vi "Simple edge timing.vi"() -> ()   [LabVIEW 2018]
uses:
  <vilib>/Platform/TimedLoop/XDataNode/timing_clust.ctl
  <vilib>/Platform/TimedLoop/XDataNode/nitl_modes.ctl
  <vilib>/Platform/TimedLoop/XDataNode/wakeup.ctl
  <vilib>/rvi/Emulation/niFpgaSctlEmulationGetInTimedLoop.vi
  <vilib>/rvi/Emulation/niFpgaProcessEmulError.vi
  <vilib>/rvi/Emulation/niFpgaEmulationReportErrorSimple.vi
  <vilib>/rvi/Emulation/niFpgaGetClockAttributes.vi
  <vilib>/rvi/Emulation/niFpgaCriticalErrorInLSC.vi
  <vilib>/rvi/eio/common/nirviEmuTemplateMethod_errors.vi
  <vilib>/platform/TimedLoop/XDataNode/XDataNode.xnode
  <vilib>/eio/EIONode/EIONode.xnode
  <vilib>/Platform/TimedLoop/XDataNode/XDNodeRunTimeDep.lvlib
panel:
  in  "STOP":bool
  out "pulses":u32 caption="Clock cycles"
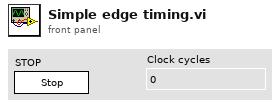
[diagram p1: front panel]
types:
  T1 = typedef "XDNodeRunTimeDep.lvlib/timing_clust.ctl" = cluster{"Expected End [f-1]":u64, "Actual End [f-1]":u64, "Finished Late? [f-1]":bool, "Expected End [i-1]":u64, "Actual End [i-1]":u64, "Finished Late? [i-1]":bool, "Expected Start [i]":u64, "Actual Start [i]":u64, "Expected Start [f]":u64, "Actual Start [f]":u64, "Source Name":string, "Structure Name":string, "Period":i64, "Deadline":i64, "Offset":i64, "Start":i64, "Priority":i32, "Timeout":i32, "Mode":T2, "Wakeup Reason":T3, "Error":errorcluster, "Source Type":string, "Secondary Source Type":string, "Global End Time":u64, "Global Start Time":u64, "Frame Duration":u64, "Iteration Duration":u64, "Assigned CPU":i32, "I/O Scan Engine Mode":u32}
  T2 = typedef "XDNodeRunTimeDep.lvlib/nitl_modes.ctl" = enum32{"No Change", "Process missed periods, maintain original phase", "Discard missed periods, maintain original phase", "Process missed periods, ignore original phase", "Discard missed periods, ignore original phase"}
  T3 = typedef "XDNodeRunTimeDep.lvlib/wakeup.ctl" = enum32{"Normal", "Aborted", "Asynchronous wakeup", "Timing source error", "Timed loop error", "Timeout"}
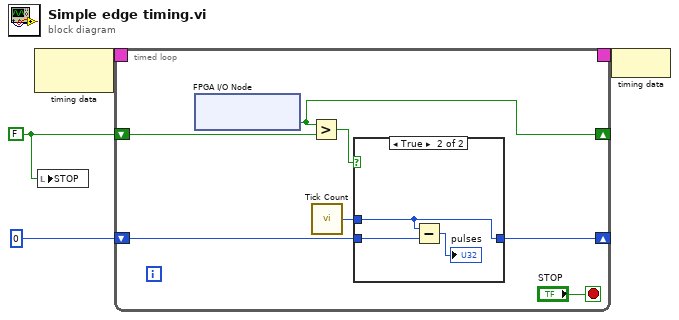
[diagram p0: block diagram]
diagram:
  w1 = FALSE
  n1 = node-c288() -> (w4:T1)  [unwired: 1 in]
  n2 = local write "STOP"(w1) -> ()
  n3 = timed-loop {
    timing: w4 -> [_]
    timing-out: [_] -> w3
    shift-right: [w9] -> _
    shift-left: w1 -> [w11]
    shift-right: [w6] -> _
    shift-left: u32 0 ("Tick Count(Ticks)") -> [w8]
    stop <- "STOP" stop-if-true
    n4 = xnode "FPGA I/O Node"() -> ("Mod8/DIO5"=w9:bool)  [unwired: 1 in, 1 out]
    n5 = Greater?(x=w9, y=w11) -> (0:w10:bool)
    n6 = call "Tick Count"() -> ("Tick Count(Ticks)"=w7:u32)
    n7 = case shown="True" w10 {
      tunnel: w8 -> [w12 w15]
      tunnel: w7 -> [_ w14]
      tunnel: [w12 w14] -> w6
      frame False {
      }
      frame True {
        n8 = Subtract(x=w14, y=w15) -> (x-y=→"pulses":u32)
      }
    }
  }
  n9 = node-c288(w3) -> ()
